vi "DAQmx测TTL信号频率.vi"() -> ()   [LabVIEW 2010]
uses:
  <vilib>/DAQmx/read.llb/DAQmx Read.vi
  <vilib>/DAQmx/read.llb/DAQmx Read (Counter 1D DBL 1Chan NSamp).vi
  <vilib>/daqmx/miscellaneous.llb/DAQmx Fill In Error Info.vi
panel:
  in  "stop":bool
  out "实测频率":dbl[](array[numeric]) caption="data" format="%0.2f"
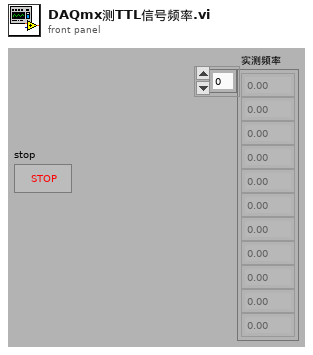
[diagram p1: front panel]
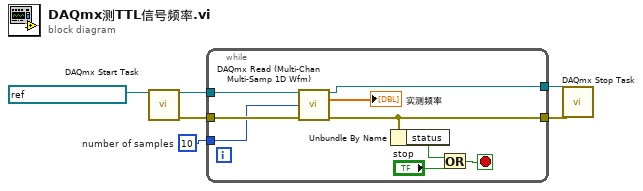
[diagram p0: block diagram]
diagram:
  w4 = 10  # number of samples
  n1 = call <vilib>:"DAQmx Start Task.vi"("task/channels in"=refnum<k21> "MyFrequencyTask") -> ("task out"=w6:refnum<k21>, "error out"=w5:errorcluster)  [unwired: 13 in]
  n2 = while {
    tunnel: w6 -> [w15]
    tunnel: w5 -> [w14]
    tunnel: w4 -> [w12]
    tunnel: [w10] -> w3
    tunnel: [w13] -> w2
    stop <- w7 stop-if-true
    n3 = call-poly "DAQmx Read (Multi-Chan Multi-Samp 1D Wfm).vi"("task/channels in"=w15, "number of samples per channel"=w12, "error in"=w14) -> ("task out"=w13:refnum<k21>, "data"=→"实测频率":dbl[], "error out"=w10:errorcluster)  [unwired: 10 in]
    n4 = Unbundle By Name(w10) -> ("status"=w8:bool)
    n5 = Or(x=w8, y="stop") -> (x .or. y?=w7:bool)
  }
  n6 = call <vilib>:"DAQmx Stop Task.vi"("task/channels in"=w2, "error in"=w3) -> ()  [unwired: 12 in, 2 out]
